vi "test_LogFile Exists on Target.vi"(8 "error in (no error)":errorcluster, 11 "TestCase in":refnum<class "Telemetry System Tests.lvclass">=refnum) -> (0 "error out":errorcluster, 3 "TestCase out":refnum<class "Telemetry System Tests.lvclass">)   [LabVIEW 2026, in "Telemetry System Tests.lvclass"]
uses:
  Telemetry System Tests.lvclass
  Telemetry System Tests.lvclass/Telemetry System Tests.ctl
  4c642fb7-04a0-4729-a002-4e235dd1b0d8.vi
  2f3db68a-3854-4bfc-845d-2781c904064a.vi
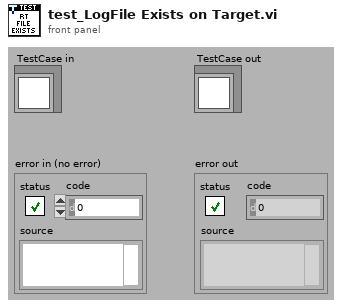
[diagram p1: front panel]
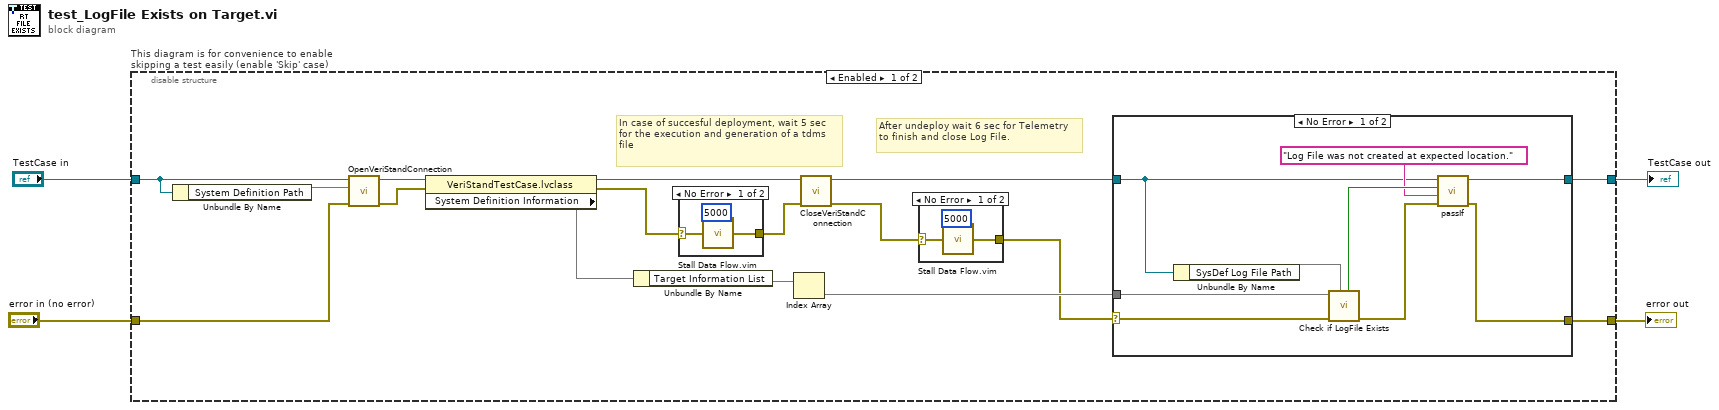
[diagram p0: block diagram]
diagram:
  n1 = disable-structure "This diagram is for convenience to enable skipping a test easily (enable 'Skip' case)" shown="Enabled" {
    disable-tunnel: "TestCase in" -> [w16 w43]
    disable-tunnel: [w19 w41] -> w1
    disable-tunnel: [w20 w42] -> w3
    disable-tunnel: "error in (no error)" -> [w17 w40]
    frame Enabled {
      # "After undeploy wait 6 sec for Telemetry to finish and close Log File."
      # "In case of succesful deployment, wait 5 sec for the execution and generation of a tdms file"
      n2 = Unbundle By Name(w16) -> ("System Definition Path"=w15)
      n3 = call-dynamic "OpenVeriStandConnection.vi"("error in (no error)"=w17, "System Definition File"=w15, "VeriStand Test Case in"=w16) -> ("error out"=w10:errorcluster, "VeriStand Test Case out"=w14:refnum<class "VeriStandTestCase.lvclass">)  [unwired: 6 in, 1 out]
      n4 = property class="VeriStandTestCase.lvclass"(reference=w14, error in=w10) -> (reference out=w13:refnum<class "VeriStandTestCase.lvclass">, error out=w8:errorcluster, "System Definition Information"=w12)
      n5 = Unbundle By Name(w12) -> ("Target Information List"=w11)
      n6 = case shown="No Error" w8 {
        selector: w8 -> [w27 w28]
        tunnel: [w25 w28] -> w7
        frame No Error {
          n7 = call "Stall Data Flow.vim"("value in"=w27, "milliseconds to wait"=u32 5000) -> ("value out"=w25:errorcluster)  [unwired: 1 out]
        }
        frame Error {
        }
      }
      n8 = Index Array(array=w11) -> (element=w9)  [unwired: 1 in]
      n9 = call-dynamic "CloseVeriStandConnection.vi"("error in (no error)"=w7, "VeriStand Test Case in"=w13) -> ("error out"=w6:errorcluster, "VeriStand Test Case out"=w18:refnum<class "VeriStandTestCase.lvclass">)  [unwired: 8 in]
      n10 = case shown="No Error" w6 {
        selector: w6 -> [w23 w24]
        tunnel: [w21 w24] -> w5
        frame No Error {
          n11 = call "Stall Data Flow.vim"("value in"=w23, "milliseconds to wait"=u32 5000) -> ("value out"=w21:errorcluster)  [unwired: 1 out]
        }
        frame Error {
        }
      }
      n12 = case shown="No Error" w5 {
        selector: w5 -> [w33 w39]
        tunnel: [w35 w39] -> w20
        tunnel: [w37 w38] -> w19
        tunnel: w18 -> [w29 w38]
        tunnel: w9 -> [w32 _]
        frame No Error {
          n13 = Unbundle By Name(w29) -> ("SysDef Log File Path"=w30)
          n14 = call "Check if LogFile Exists.vi"("Log File Path"=w30, "error in (no error)"=w33, "Target Information"=w32) -> ("error out"=w36:errorcluster, "LogFile Exists?"=w34:bool)  [unwired: 6 in, 1 out]
          n15 = call-dynamic "passIf.vi"("error in (no error)"=w36, "message (\"\")"="Log File was not created at expected location." ("message (\"\")"), "pass"=w34, "TestCase in"=w29) -> ("error out"=w35:errorcluster, "TestCase out"=w37:refnum<class "Telemetry System Tests.lvclass">)  [unwired: 6 in]
        }
        frame Error {
        }
      }
    }
    frame Disabled {
      # "skip test result while test is under development"
      n16 = call <vilib>:"skip.vi"("error in (no error)"=w40, "TestCase in"=w43) -> ("error out"=w42:errorcluster, "TestCase out"=w41:refnum<class "Telemetry System Tests.lvclass">)  [unwired: 8 in]
    }
  }
  "error out" <- w3
  "TestCase out" <- w1
